vi "WPI_CANTalonSRX_Global.vi"(6 "Set Boolean":bool, 7 "Write After Receive":T2, 8 "Set Number":dbl, 9 "Control Mode":T1, 10 "Operation":T7, 11 "Device ID (0)":u8) -> (1 "Get All":T2, 3 "Device ID Out":u8, 5 "Read For Send":T3={"Output"=0.0, "Control Mode"=enum."Percent VBus", "Brake-Mode Override"=enum."No Override", "Reverse Feedback Sensor"=FALSE, "Reverse Closed-Loop Output"=FALSE, "Override Limits"=FALSE, "Forward Limit Enabled"=FALSE, "Reverse Limit Enabled"=FALSE, "Feedback Select"=0, "Profile Select"=0, "Master To Follow"=0, "Throttle Ramp Rate"=0, "Disabled"=FALSE, "Encoder Codes Per Rev"=0, "Num Pot Turns"=0, "Control Frame Rate Ms"=0, "Use Control5 If Supported"=FALSE, "Enable Frame Rate Ms"=10, "Motion Profile Flow Control"=0, "Motion Profile Control Frame Rate"=10, "Talon SRX Motion Profile Trajectory Point"={"Duration Ms"=0, "Velocity"=0.0, "Position"=0.0, "Profile Slot Select"=0, "Is Last"=FALSE, "Velocity Only"=FALSE, "Zero Position"=FALSE, "Compress Code"=0, "Same Velocity"=0, "Delta Position"=0, "Count"=0}, "Current Limit Enabled"=FALSE} {"Feedback Select" items=["Digital Quadrature Encoder"=0, "Analog Pot"=2, "Analog Encoder"=3, "Count on Quad-A (Rising-Edge)"=4, "Count on Quad-A (Falling-Edge)"=5, "Position is Pulse-Width"=8, "CTR Magnetic Enc (Relative)"=6, "CTR Magnetic Enc (Absolute)"=7]})   [LabVIEW 2016]
uses:
  WPI_CANTalonSRX_GlobalOps.ctl
  WPI_CANTalonSRX_GlobalControl.ctl
  WPI_CANTalonSRX_APIControlMode.ctl
  WPI_CANTalonSRX_BrakeOverride.ctl
  WPI_CANTalonSRX_FeedbackSelect.ctl
  WPI_CANTalonSRX_MotionProfileTrajectoryPt.ctl
  WPI_CANTalonSRX_GlobalStatus.ctl
  WPI_CANTalonSRX_MessageIDs.ctl
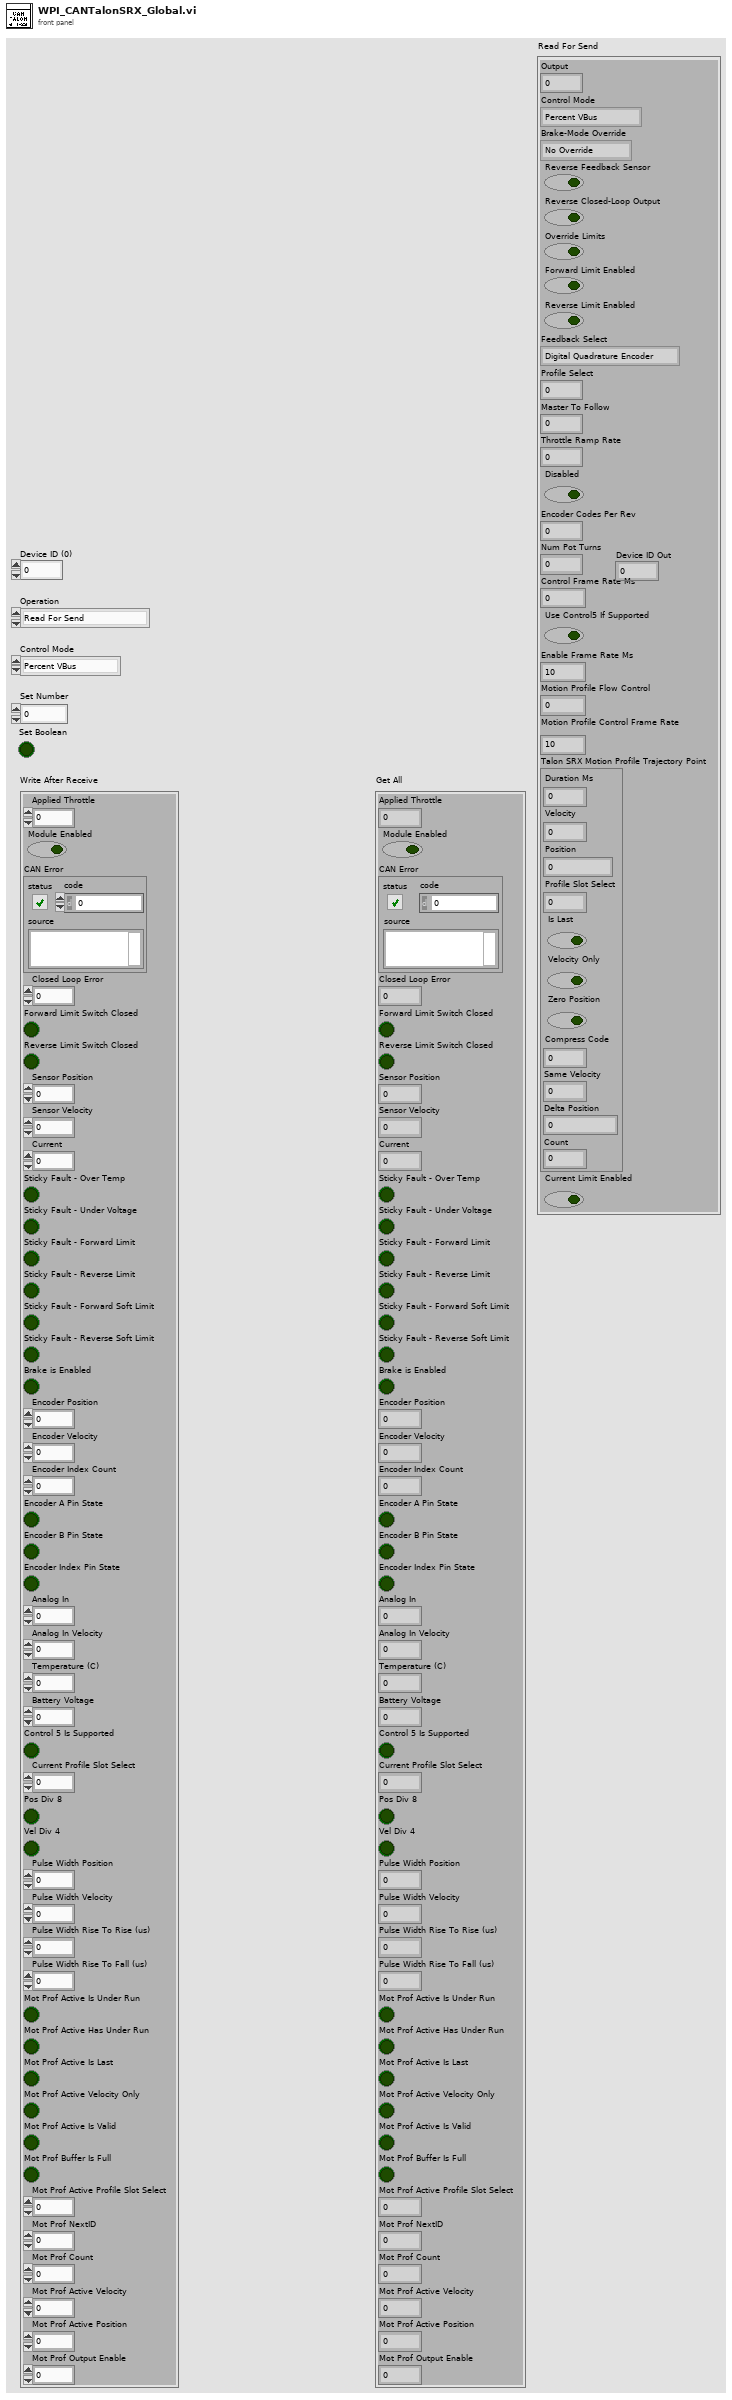
[diagram p1: front panel]
types:
  T1 = typedef "WPI_CANTalonSRX_APIControlMode.ctl" = enum8{"Percent VBus", "Speed", "Position", "Slave", "Unchanged / Invalid", "Voltage Compensation", "Current", "Motion Profile", "Motion Magic"}
  T2 = typedef "WPI_CANTalonSRX_GlobalStatus.ctl" = cluster{"Applied Throttle":dbl, "Module Enabled":bool, "CAN Error":errorcluster, "Closed Loop Error":dbl, "Forward Limit Switch Closed":bool, "Reverse Limit Switch Closed":bool, "Sensor Position":dbl, "Sensor Velocity":dbl, "Current":dbl, "Sticky Fault - Over Temp":bool, "Sticky Fault - Under Voltage":bool, "Sticky Fault - Forward Limit":bool, "Sticky Fault - Reverse Limit":bool, "Sticky Fault - Forward Soft Limit":bool, "Sticky Fault - Reverse Soft Limit":bool, "Brake is Enabled":bool, "Encoder Position":dbl, "Encoder Velocity":dbl, "Encoder Index Count":dbl, "Encoder A Pin State":bool, "Encoder B Pin State":bool, "Encoder Index Pin State":bool, "Analog In":dbl, "Analog In Velocity":dbl, "Temperature (C)":dbl, "Battery Voltage":dbl, "Control 5 Is Supported":bool, "Current Profile Slot Select":dbl, "Pos Div 8":bool, "Vel Div 4":bool, "Pulse Width Position":i32, "Pulse Width Velocity":i32, "Pulse Width Rise To Rise (us)":i32, "Pulse Width Rise To Fall (us)":i32, "Mot Prof Active Is Under Run":bool, "Mot Prof Active Has Under Run":bool, "Mot Prof Active Is Last":bool, "Mot Prof Active Velocity Only":bool, "Mot Prof Active Is Valid":bool, "Mot Prof Buffer Is Full":bool, "Mot Prof Active Profile Slot Select":i32, "Mot Prof NextID":i32, "Mot Prof Count":i32, "Mot Prof Active Velocity":dbl, "Mot Prof Active Position":dbl, "Mot Prof Output Enable":i32}
  T3 = typedef "WPI_CANTalonSRX_GlobalControl.ctl" = cluster{"Output":dbl, "Control Mode":T1, "Brake-Mode Override":T4, "Reverse Feedback Sensor":bool, "Reverse Closed-Loop Output":bool, "Override Limits":bool, "Forward Limit Enabled":bool, "Reverse Limit Enabled":bool, "Feedback Select":T5, "Profile Select":u8, "Master To Follow":u8, "Throttle Ramp Rate":u8, "Disabled":bool, "Encoder Codes Per Rev":u32, "Num Pot Turns":u32, "Control Frame Rate Ms":u8, "Use Control5 If Supported":bool, "Enable Frame Rate Ms":u8, "Motion Profile Flow Control":u8, "Motion Profile Control Frame Rate":u8, "Talon SRX Motion Profile Trajectory Point":T6, "Current Limit Enabled":bool}
  T4 = typedef "WPI_CANTalonSRX_BrakeOverride.ctl" = enum8{"No Override", "Override to Coast", "Override to Brake"}
  T5 = typedef "WPI_CANTalonSRX_FeedbackSelect.ctl" = u8
  T6 = typedef "WPI_CANTalonSRX_MotionProfileTrajectoryPt.ctl" = cluster{"Duration Ms":u8, "Velocity":dbl, "Position":dbl, "Profile Slot Select":u8, "Is Last":bool, "Velocity Only":bool, "Zero Position":bool, "Compress Code":u8, "Same Velocity":i32, "Delta Position":i32, "Count":u8}
  T7 = typedef "WPI_CANTalonSRX_GlobalOps.ctl" = enum16{"Read For Send", "Write After Receive General", "Write After Receive Feedback", "Write After Receive Encoder", "Write After Receive Ain", "Write Error", "Get All", "Set Output", "Set Mode", "Set Master ID", "Set Brake Mode", "Set Reverse Feedback Sensor", "Set Reverse Closed Loop Output", "Set Override Limits", "Set Forward Limit Enabled", "Set Reverse Limit Enabled", "Set Feedback Select", "Set Profile Select", "Set Throttle Ramp Rate", "Disable", "Set Enc Codes Per Rev", "Set Num Pot Turns", "Set Control Frame Rate", "Enable Legacy Control", "Write After Receive Pulse Width", "Set Enable Frame Rate", "Write After Receive Motion Profile", "Set Motion Profile Flow Control", "Set Motion Profile Control Frame Rate", "Set Current Limit Enable"}
  T8 = typedef "WPI_CANTalonSRX_MessageIDs.ctl" = u32
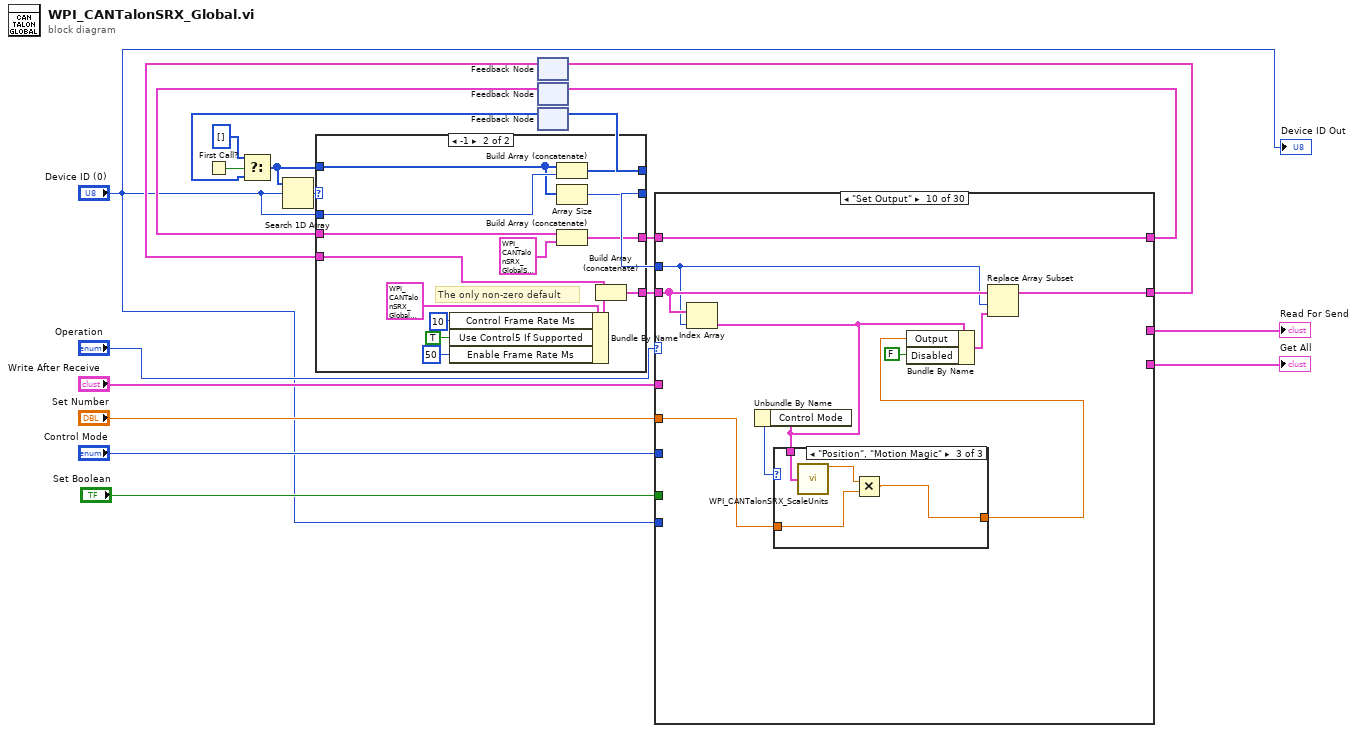
[diagram p0: block diagram]
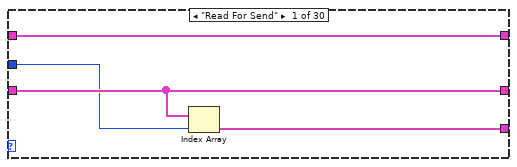
[diagram p2: hidden frame]
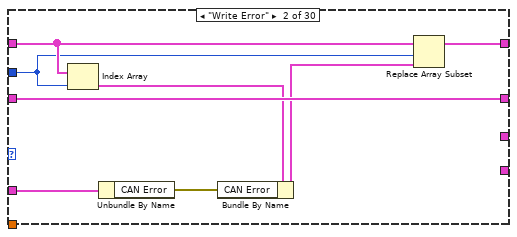
[diagram p3: hidden frame]
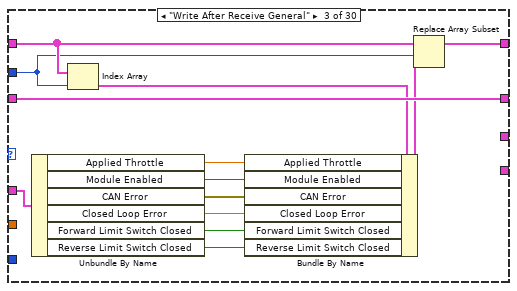
[diagram p4: hidden frame]
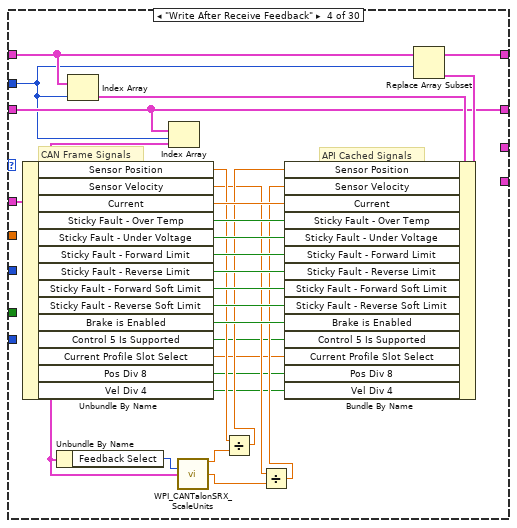
[diagram p5: hidden frame]
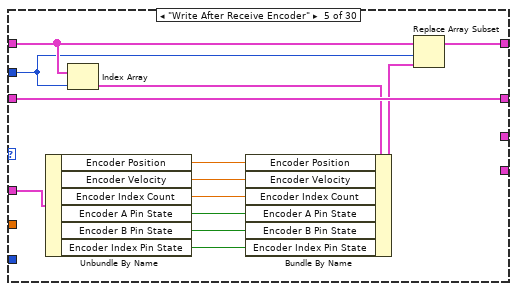
[diagram p6: hidden frame]
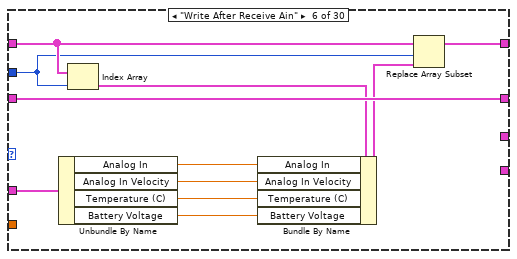
[diagram p7: hidden frame]
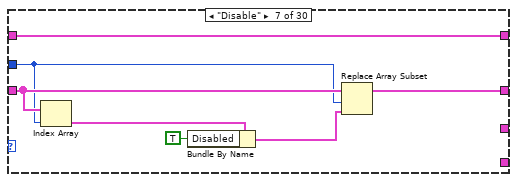
[diagram p8: hidden frame]
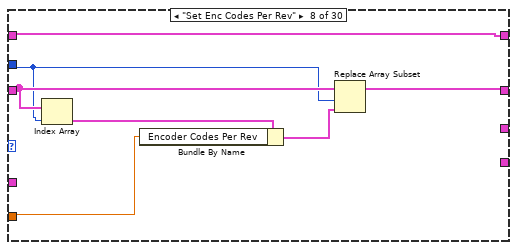
[diagram p9: hidden frame]
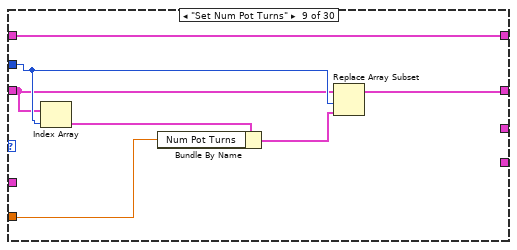
[diagram p10: hidden frame]
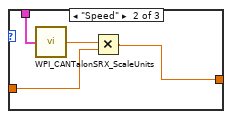
[diagram p12: hidden frame]
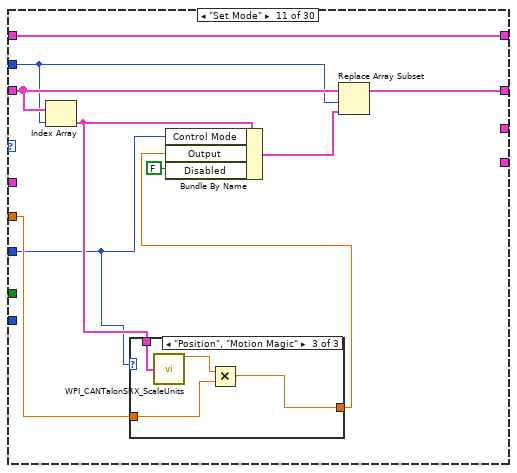
[diagram p13: hidden frame]
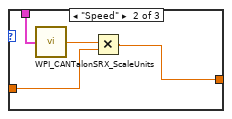
[diagram p15: hidden frame]
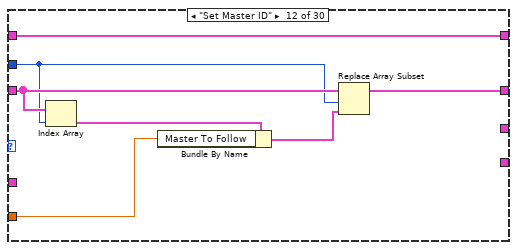
[diagram p16: hidden frame]
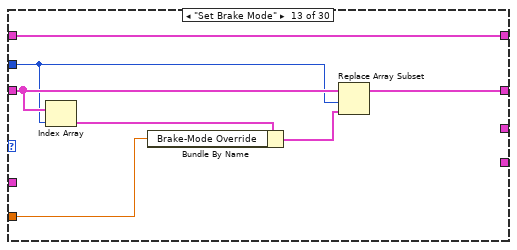
[diagram p17: hidden frame]
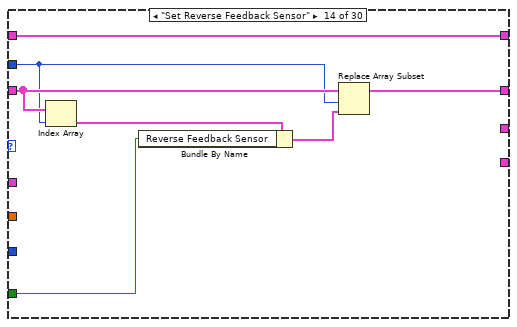
[diagram p18: hidden frame]
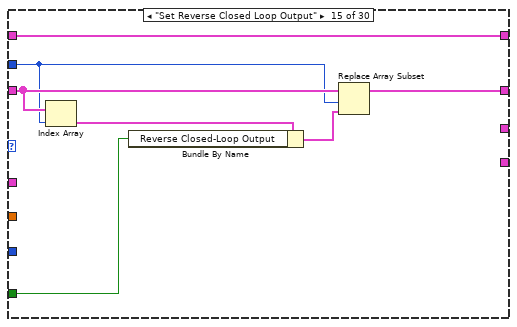
[diagram p19: hidden frame]
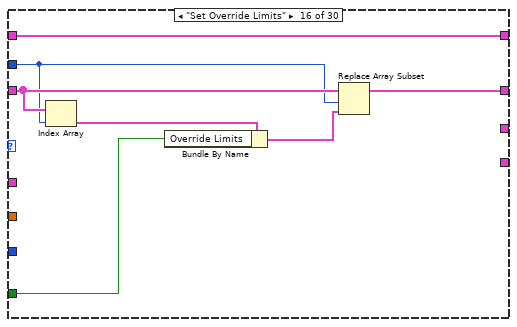
[diagram p20: hidden frame]
diagram:
  n1 = First Call?() -> (First Call?: T/F=w21:bool)
  n2 = feedback #1() -> (w14:T3[])  [unwired: 1 in]
  n3 = feedback #2() -> (w15:T2[])  [unwired: 1 in]
  n4 = feedback #3() -> (w19:u8[])  [unwired: 1 in]
  n5 = Select(t=u8[] [], s=w21, f=w19) -> (s? t:f=w17:u8[])
  n6 = Search 1D Array(1D array=w17, element="Device ID (0)") -> (index of element=w16:i32)  [unwired: 1 in]
  n7 = case shown="-1" w16 {
    selector: w16 -> [w22 _]
    tunnel: [w25 w39] -> w18
    tunnel: "Device ID (0)" -> [_ w38]
    tunnel: w17 -> [w25 w33]
    tunnel: w15 -> [w24 w37]
    tunnel: w14 -> [w23 w36]
    tunnel: [w24 w35] -> w12
    tunnel: [w23 w34] -> w10
    tunnel: [w22 w32] -> w9
    frame Default {
    }
    frame -1 {
      # "The only non-zero default"
      n8 = Bundle By Name(cluster=T3 {"Output"=0.0, "Control Mode"=enum."Percent VBus", "Brake-Mode Override"=enum."No Override", "Reverse Feedback Sensor"=FALSE, "Reverse Closed-Loop Output"=FALSE, "Override Limits"=FALSE, "Forward Limit Enabled"=FALSE, "Reverse Limit Enabled"=FALSE, "Feedback Select"=0, "Profile Select"=0, "Master To Follow"=0, "Throttle Ramp Rate"=0, "Disabled"=FALSE, "Encoder Codes Per Rev"=0, "Num Pot Turns"=0, "Control Frame Rate Ms"=0, "Use Control5 If Supported"=FALSE, "Enable Frame Rate Ms"=10, "Motion Profile Flow Control"=0, "Motion Profile Control Frame Rate"=10, "Talon SRX Motion Profile Trajectory Point"={"Duration Ms"=0, "Velocity"=0.0, "Position"=0.0, "Profile Slot Select"=0, "Is Last"=FALSE, "Velocity Only"=FALSE, "Zero Position"=FALSE, "Compress Code"=0, "Same Velocity"=0, "Delta Position"=0, "Count"=0}, "Current Limit Enabled"=FALSE} ("Read For Send"), "Control Frame Rate Ms"=u8 10, "Use Control5 If Supported"=TRUE, "Enable Frame Rate Ms"=u8 50) -> (w30:T3)
      n9 = Build Array (concatenate)(w33, w38) -> (w39:u8[])
      n10 = Array Size(array=w33) -> (size(s)=w32:i32)
      n11 = Build Array (concatenate)(w37, T2 {"Applied Throttle"=0.0, "Module Enabled"=FALSE, "CAN Error"={"status"=FALSE, "code"=0, "source"=""}, "Closed Loop Error"=0.0, "Forward Limit Switch Closed"=FALSE, "Reverse Limit Switch Closed"=FALSE, "Sensor Position"=0.0, "Sensor Velocity"=0.0, "Current"=0.0, "Sticky Fault - Over Temp"=FALSE, "Sticky Fault - Under Voltage"=FALSE, "Sticky Fault - Forward Limit"=FALSE, "Sticky Fault - Reverse Limit"=FALSE, "Sticky Fault - Forward Soft Limit"=FALSE, "Sticky Fault - Reverse Soft Limit"=FALSE, "Brake is Enabled"=FALSE, "Encoder Position"=0.0, "Encoder Velocity"=0.0, "Encoder Index Count"=0.0, "Encoder A Pin State"=FALSE, "Encoder B Pin State"=FALSE, "Encoder Index Pin State"=FALSE, "Analog In"=0.0, "Analog In Velocity"=0.0, "Temperature (C)"=0.0, "Battery Voltage"=0.0, "Control 5 Is Supported"=FALSE, "Current Profile Slot Select"=0.0, "Pos Div 8"=FALSE, "Vel Div 4"=FALSE, "Pulse Width Position"=0, "Pulse Width Velocity"=0, "Pulse Width Rise To Rise (us)"=0, "Pulse Width Rise To Fall (us)"=0, "Mot Prof Active Is Under Run"=FALSE, "Mot Prof Active Has Under Run"=FALSE, "Mot Prof Active Is Last"=FALSE, "Mot Prof Active Velocity Only"=FALSE, "Mot Prof Active Is Valid"=FALSE, "Mot Prof Buffer Is Full"=FALSE, "Mot Prof Active Profile Slot Select"=0, "Mot Prof NextID"=0, "Mot Prof Count"=0, "Mot Prof Active Velocity"=0.0, "Mot Prof Active Position"=0.0, "Mot Prof Output Enable"=0} ("Write After Receive")) -> (w35:T2[])
      n12 = Build Array (concatenate)(w36, w30) -> (w34:T3[])
    }
  }
  n13 = feedback-in #3(w18) -> ()
  n14 = case shown="\"Set Output\"" "Operation" {
    tunnel: [w43 w50 w63 w91 w103 w114 w122 w128 w130 w146 w161 w176 w183 w190 w197 w204 w211 w218 w225 w232 w239 w246 w252 w264 w273 w283 w306 w320 w324 w335] -> w13
    tunnel: w12 -> [w43 w49 w62 w90 w102 w113 w122 w128 w130 w146 w161 w176 w183 w190 w197 w204 w211 w218 w225 w232 w239 w246 w252 w264 w274 w283 w307 w320 w324 w335]
    tunnel: [w42 w51 w64 w78 w104 w115 w120 w125 w133 w144 w165 w181 w188 w195 w202 w209 w216 w223 w230 w237 w244 w248 w254 w261 w272 w282 w296 w319 w323 w332] -> w11
    tunnel: w10 -> [w42 w51 w64 w78 w104 w115 w121 w127 w131 w145 w164 w180 w187 w194 w201 w208 w215 w222 w229 w236 w243 w248 w255 w262 w272 w284 w296 w317 w326 w333]
    tunnel: w9 -> [w41 w48 w61 w77 w101 w112 w119 w124 w132 w143 w163 w179 w186 w193 w200 w207 w214 w221 w228 w235 w242 w247 w253 w263 w275 w285 w295 w321 w325 w334]
    tunnel: [w40 _ _ _ _ _ _ _ _ _ _ _ _ _ _ _ _ _ _ _ _ _ _ _ _ _ _ _ _ _] -> w8
    tunnel: "Write After Receive" -> [_ w45 w60 w89 w100 w111 _ _ _ _ _ _ _ _ _ _ _ _ _ _ _ _ _ _ w271 _ w308 _ _ _]
    tunnel: "Set Number" -> [_ _ _ _ _ _ _ w126 w134 w139 w159 w175 w182 _ _ _ _ _ w224 w231 w238 _ w250 _ _ w286 _ w316 w327 _]
    tunnel: [_ _ _ _ _ _ _ _ _ _ _ _ _ _ _ _ _ _ _ _ _ w245 _ _ _ _ _ _ _ _] -> w5
    tunnel: "Control Mode" -> [_ _ _ _ _ _ _ _ _ _ w156 _ _ _ _ _ _ _ _ _ _ _ _ _ _ _ _ _ _ _]
    tunnel: "Set Boolean" -> [_ _ _ _ _ _ _ _ _ _ _ _ _ w189 w196 w203 w210 w217 _ _ _ _ _ w258 _ _ _ _ _ w331]
    tunnel: "Device ID (0)" -> [_ _ _ _ _ _ _ _ _ _ _ _ _ _ _ _ _ _ _ _ _ _ _ w259 _ _ _ _ _ _]
    frame "Read For Send" {
      n15 = Index Array(array=w42, index=w41) -> (element=w40:T3)
    }
    frame "Write Error" {
      n16 = Index Array(array=w49, index=w48) -> (element=w47:T2)
      n17 = Unbundle By Name(w45) -> ("CAN Error"=w44:errorcluster)
      n18 = Bundle By Name(cluster=w47, "CAN Error"=w44) -> (w46:T2)
      n19 = Replace Array Subset(array=w49, new element=w46, index=w48) -> (w50:T2[])
    }
    frame "Write After Receive General" {
      n20 = Unbundle By Name(w60) -> ("Applied Throttle"=w57:dbl, "Module Enabled"=w56:bool, "CAN Error"=w55:errorcluster, "Closed Loop Error"=w54:dbl, "Forward Limit Switch Closed"=w53:bool, "Reverse Limit Switch Closed"=w52:bool)
      n21 = Index Array(array=w62, index=w61) -> (element=w59:T2)
      n22 = Bundle By Name(cluster=w59, "Applied Throttle"=w57, "Module Enabled"=w56, "CAN Error"=w55, "Closed Loop Error"=w54, "Forward Limit Switch Closed"=w53, "Reverse Limit Switch Closed"=w52) -> (w58:T2)
      n23 = Replace Array Subset(array=w62, new element=w58, index=w61) -> (w63:T2[])
    }
    frame "Write After Receive Feedback" {
      # "API Cached Signals"
      # "CAN Frame Signals"
      n24 = Unbundle By Name(w89) -> ("Sensor Position"=w75:dbl, "Sensor Velocity"=w73:dbl, "Current"=w86:dbl, "Sticky Fault - Over Temp"=w85:bool, "Sticky Fault - Under Voltage"=w84:bool, "Sticky Fault - Forward Limit"=w83:bool, "Sticky Fault - Reverse Limit"=w79:bool, "Sticky Fault - Forward Soft Limit"=w80:bool, "Sticky Fault - Reverse Soft Limit"=w81:bool, "Brake is Enabled"=w82:bool, "Control 5 Is Supported"=w65:bool, "Current Profile Slot Select"=w66:dbl, "Pos Div 8"=w67:bool, "Vel Div 4"=w68:bool)
      n25 = Index Array(array=w90, index=w77) -> (element=w88:T2)
      n26 = Index Array(array=w78, index=w77) -> (element=w70:T3)
      n27 = Unbundle By Name(w70) -> ("Feedback Select"=w69:T5)
      n28 = call "WPI_CANTalonSRX_ScaleUnits.vi"("Feedback Scalar Select"=w69, "Read For Send"=w70) -> ("Position Scalar"=w74:dbl, "Velocity Scalar"=w72:dbl)  [unwired: 11 in, 1 out]
      n29 = Divide(x=w75, y=w74) -> (x/y=w76:dbl)
      n30 = Divide(x=w73, y=w72) -> (x/y=w71:dbl)
      n31 = Bundle By Name(cluster=w88, "Sensor Position"=w76, "Sensor Velocity"=w71, "Current"=w86, "Sticky Fault - Over Temp"=w85, "Sticky Fault - Under Voltage"=w84, "Sticky Fault - Forward Limit"=w83, "Sticky Fault - Reverse Limit"=w79, "Sticky Fault - Forward Soft Limit"=w80, "Sticky Fault - Reverse Soft Limit"=w81, "Brake is Enabled"=w82, "Control 5 Is Supported"=w65, "Current Profile Slot Select"=w66, "Pos Div 8"=w67, "Vel Div 4"=w68) -> (w87:T2)
      n32 = Replace Array Subset(array=w90, new element=w87, index=w77) -> (w91:T2[])
    }
    frame "Write After Receive Encoder" {
      n33 = Unbundle By Name(w100) -> ("Encoder Position"=w97:dbl, "Encoder Velocity"=w96:dbl, "Encoder Index Count"=w95:dbl, "Encoder A Pin State"=w94:bool, "Encoder B Pin State"=w93:bool, "Encoder Index Pin State"=w92:bool)
      n34 = Index Array(array=w102, index=w101) -> (element=w99:T2)
      n35 = Bundle By Name(cluster=w99, "Encoder Position"=w97, "Encoder Velocity"=w96, "Encoder Index Count"=w95, "Encoder A Pin State"=w94, "Encoder B Pin State"=w93, "Encoder Index Pin State"=w92) -> (w98:T2)
      n36 = Replace Array Subset(array=w102, new element=w98, index=w101) -> (w103:T2[])
    }
    frame "Write After Receive Ain" {
      n37 = Unbundle By Name(w111) -> ("Analog In"=w108:dbl, "Analog In Velocity"=w107:dbl, "Temperature (C)"=w106:dbl, "Battery Voltage"=w105:dbl)
      n38 = Index Array(array=w113, index=w112) -> (element=w110:T2)
      n39 = Bundle By Name(cluster=w110, "Analog In"=w108, "Analog In Velocity"=w107, "Temperature (C)"=w106, "Battery Voltage"=w105) -> (w109:T2)
      n40 = Replace Array Subset(array=w113, new element=w109, index=w112) -> (w114:T2[])
    }
    frame "Disable" {
      n41 = Index Array(array=w121, index=w119) -> (element=w118:T3)
      n42 = Bundle By Name(cluster=w118, "Disabled"=TRUE) -> (w117:T3)
      n43 = Replace Array Subset(array=w121, new element=w117, index=w119) -> (w120:T3[])
    }
    frame "Set Enc Codes Per Rev" {
      n44 = Index Array(array=w127, index=w124) -> (element=w123:T3)
      n45 = Bundle By Name(cluster=w123, "Encoder Codes Per Rev"=w126) -> (w129:T3)
      n46 = Replace Array Subset(array=w127, new element=w129, index=w124) -> (w125:T3[])
    }
    frame "Set Num Pot Turns" {
      n47 = Index Array(array=w131, index=w132) -> (element=w135:T3)
      n48 = Bundle By Name(cluster=w135, "Num Pot Turns"=w134) -> (w136:T3)
      n49 = Replace Array Subset(array=w131, new element=w136, index=w132) -> (w133:T3[])
    }
    frame "Set Output" {
      n50 = Index Array(array=w145, index=w143) -> (element=w137:T3)
      n51 = Unbundle By Name(w137) -> ("Control Mode"=w140:T1)
      n52 = case shown="\"Position\", \"Motion Magic\"" w140 {
        tunnel: [w147 w148 w154] -> w138
        tunnel: w139 -> [w147 w150 w152]
        tunnel: w137 -> [_ w151 w155]
        frame Default {
        }
        frame "Speed" {
          n53 = call "WPI_CANTalonSRX_ScaleUnits.vi"("Read For Send"=w151) -> ("Velocity Scalar"=w149:dbl)  [unwired: 12 in, 2 out]
          n54 = Multiply(x=w149, y=w150) -> (x*y=w148:dbl)
        }
        frame "Position", "Motion Magic" {
          n55 = call "WPI_CANTalonSRX_ScaleUnits.vi"("Read For Send"=w155) -> ("Position Scalar"=w153:dbl)  [unwired: 12 in, 2 out]
          n56 = Multiply(x=w153, y=w152) -> (x*y=w154:dbl)
        }
      }
      n57 = Bundle By Name(cluster=w137, "Output"=w138, "Disabled"=FALSE) -> (w142:T3)
      n58 = Replace Array Subset(array=w145, new element=w142, index=w143) -> (w144:T3[])
    }
    frame "Set Mode" {
      n59 = Index Array(array=w164, index=w163) -> (element=w157:T3)
      n60 = case shown="\"Position\", \"Motion Magic\"" w156 {
        tunnel: [w166 w167 w173] -> w158
        tunnel: w159 -> [w166 w169 w171]
        tunnel: w157 -> [_ w170 w174]
        frame Default {
        }
        frame "Speed" {
          n61 = call "WPI_CANTalonSRX_ScaleUnits.vi"("Read For Send"=w170) -> ("Velocity Scalar"=w168:dbl)  [unwired: 12 in, 2 out]
          n62 = Multiply(x=w168, y=w169) -> (x*y=w167:dbl)
        }
        frame "Position", "Motion Magic" {
          n63 = call "WPI_CANTalonSRX_ScaleUnits.vi"("Read For Send"=w174) -> ("Position Scalar"=w172:dbl)  [unwired: 12 in, 2 out]
          n64 = Multiply(x=w172, y=w171) -> (x*y=w173:dbl)
        }
      }
      n65 = Bundle By Name(cluster=w157, "Control Mode"=w156, "Output"=w158, "Disabled"=FALSE) -> (w162:T3)
      n66 = Replace Array Subset(array=w164, new element=w162, index=w163) -> (w165:T3[])
    }
    frame "Set Master ID" {
      n67 = Index Array(array=w180, index=w179) -> (element=w178:T3)
      n68 = Bundle By Name(cluster=w178, "Master To Follow"=w175) -> (w177:T3)
      n69 = Replace Array Subset(array=w180, new element=w177, index=w179) -> (w181:T3[])
    }
    frame "Set Brake Mode" {
      n70 = Index Array(array=w187, index=w186) -> (element=w185:T3)
      n71 = Bundle By Name(cluster=w185, "Brake-Mode Override"=w182) -> (w184:T3)
      n72 = Replace Array Subset(array=w187, new element=w184, index=w186) -> (w188:T3[])
    }
    frame "Set Reverse Feedback Sensor" {
      n73 = Index Array(array=w194, index=w193) -> (element=w192:T3)
      n74 = Bundle By Name(cluster=w192, "Reverse Feedback Sensor"=w189) -> (w191:T3)
      n75 = Replace Array Subset(array=w194, new element=w191, index=w193) -> (w195:T3[])
    }
    frame "Set Reverse Closed Loop Output" {
      n76 = Index Array(array=w201, index=w200) -> (element=w199:T3)
      n77 = Bundle By Name(cluster=w199, "Reverse Closed-Loop Output"=w196) -> (w198:T3)
      n78 = Replace Array Subset(array=w201, new element=w198, index=w200) -> (w202:T3[])
    }
    frame "Set Override Limits" {
      n79 = Index Array(array=w208, index=w207) -> (element=w206:T3)
      n80 = Bundle By Name(cluster=w206, "Override Limits"=w203) -> (w205:T3)
      n81 = Replace Array Subset(array=w208, new element=w205, index=w207) -> (w209:T3[])
    }
    frame "Set Forward Limit Enabled" {
      n82 = Index Array(array=w215, index=w214) -> (element=w213:T3)
      n83 = Bundle By Name(cluster=w213, "Forward Limit Enabled"=w210) -> (w212:T3)
      n84 = Replace Array Subset(array=w215, new element=w212, index=w214) -> (w216:T3[])
    }
    frame "Set Reverse Limit Enabled" {
      n85 = Index Array(array=w222, index=w221) -> (element=w220:T3)
      n86 = Bundle By Name(cluster=w220, "Reverse Limit Enabled"=w217) -> (w219:T3)
      n87 = Replace Array Subset(array=w222, new element=w219, index=w221) -> (w223:T3[])
    }
    frame "Set Feedback Select" {
      n88 = Index Array(array=w229, index=w228) -> (element=w227:T3)
      n89 = Bundle By Name(cluster=w227, "Feedback Select"=w224) -> (w226:T3)
      n90 = Replace Array Subset(array=w229, new element=w226, index=w228) -> (w230:T3[])
    }
    frame "Set Profile Select" {
      n91 = Index Array(array=w236, index=w235) -> (element=w234:T3)
      n92 = Bundle By Name(cluster=w234, "Profile Select"=w231) -> (w233:T3)
      n93 = Replace Array Subset(array=w236, new element=w233, index=w235) -> (w237:T3[])
    }
    frame "Set Throttle Ramp Rate" {
      n94 = Index Array(array=w243, index=w242) -> (element=w241:T3)
      n95 = Bundle By Name(cluster=w241, "Throttle Ramp Rate"=w238) -> (w240:T3)
      n96 = Replace Array Subset(array=w243, new element=w240, index=w242) -> (w244:T3[])
    }
    frame "Get All" {
      n97 = Index Array(array=w246, index=w247) -> (element=w245:T2)
    }
    frame "Set Control Frame Rate" {
      n98 = Index Array(array=w255, index=w253) -> (element=w251:T3)
      n99 = To Unsigned Byte Integer(number=w250) -> (unsigned 8bit integer=w249:u8)
      n100 = Bundle By Name(cluster=w251, "Control Frame Rate Ms"=w249) -> (w256:T3)
      n101 = Replace Array Subset(array=w255, new element=w256, index=w253) -> (w254:T3[])
    }
    frame "Enable Legacy Control" {
      n102 = Index Array(array=w262, index=w263) -> (element=w265:T3)
      n103 = case shown="True" w258 {
        tunnel: w259 -> [_ w266]
        frame False {
        }
        frame True {
          w267 = T8 33816832 items=["TalonSRX Control General 10ms"=33816576, "TalonSRX Control Rates Slow"=33816640, "TalonSRX Control ClearFlags Slow"=33816704, "TalonSRX Status General 10ms"=33821696, "TalonSRX Status Feedback 20ms"=33821760, "TalonSRX Status Enc 100ms"=33821824, "TalonSRX Status AinTempVbat 100ms"=33821888, "TalonSRX Status Startup Once"=33821952, "TalonSRX Status Debug"=33822080, "TalonSRX Config SetGainsSlot0 A"=33823808, "TalonSRX Config SetGainsSlot0 B"=33823872, "TalonSRX Config SetGainsSlot1 A"=33823936, "TalonSRX Config SetGainsSlot1 B"=33824000, "TalonSRX Config SetSoftLimits"=33824064, "TalonSRX Config WebControl"=33824128, "TalonSRX Param Request"=33822720, "TalonSRX Param Response"=33822784, "TalonSRX Param Set"=33822848, "TalonSRX Status PulseWidth"=33822144, "TalonSRX Status Motion Profile"=33822208, "TalonSRX Control General 5"=33816832, "TalonSRX Control Motion Profile Add"=33816896] ("Talon SRX Control Frame")
          # "Turn off Control 5, Send VI will use Control 1"
          n104 = Or(x=w266, y=w267) -> (x .or. y?=w268:T8)
          n105 = call <vilib>:"NetComm_CAN_Send.vi"("Period (ms)"=0, "Data"=u8[] [] ("Token Space"), "Message ID"=w268) -> ()  [unwired: 8 in, 1 out]
        }
      }
      n106 = Not(x=w258) -> (.not. x?=w260:bool)
      n107 = Bundle By Name(cluster=w265, "Use Control5 If Supported"=w260) -> (w257:T3)
      n108 = Replace Array Subset(array=w262, new element=w257, index=w263) -> (w261:T3[])
    }
    frame "Write After Receive Pulse Width" {
      n109 = Unbundle By Name(w271) -> ("Pulse Width Position"=w279:i32, "Pulse Width Velocity"=w278:i32, "Pulse Width Rise To Rise (us)"=w277:i32, "Pulse Width Rise To Fall (us)"=w276:i32)
      n110 = Index Array(array=w274, index=w275) -> (element=w281:T2)
      n111 = Bundle By Name(cluster=w281, "Pulse Width Position"=w279, "Pulse Width Velocity"=w278, "Pulse Width Rise To Rise (us)"=w277, "Pulse Width Rise To Fall (us)"=w276) -> (w280:T2)
      n112 = Replace Array Subset(array=w274, new element=w280, index=w275) -> (w273:T2[])
    }
    frame "Set Enable Frame Rate" {
      n113 = Index Array(array=w284, index=w285) -> (element=w288:T3)
      n114 = To Unsigned Byte Integer(number=w286) -> (unsigned 8bit integer=w287:u8)
      n115 = Bundle By Name(cluster=w288, "Enable Frame Rate Ms"=w287) -> (w289:T3)
      n116 = Replace Array Subset(array=w284, new element=w289, index=w285) -> (w282:T3[])
    }
    frame "Write After Receive Motion Profile" {
      # "API Cached Signals"
      # "CAN Frame Signals"
      n117 = Unbundle By Name(w308) -> ("Mot Prof Active Is Under Run"=w312:bool, "Mot Prof Active Has Under Run"=w311:bool, "Mot Prof Active Is Last"=w310:bool, "Mot Prof Active Velocity Only"=w309:bool, "Mot Prof Active Is Valid"=w305:bool, "Mot Prof Buffer Is Full"=w304:bool, "Mot Prof Active Profile Slot Select"=w303:i32, "Mot Prof NextID"=w302:i32, "Mot Prof Count"=w301:i32, "Mot Prof Active Velocity"=w293:dbl, "Mot Prof Active Position"=w291:dbl, "Mot Prof Output Enable"=w300:i32)
      n118 = Index Array(array=w296, index=w295) -> (element=w294:T3)
      n119 = Unbundle By Name(w294) -> ("Feedback Select"=w297:T5)
      n120 = Index Array(array=w307, index=w295) -> (element=w314:T2)
      n121 = call "WPI_CANTalonSRX_ScaleUnits.vi"("Feedback Scalar Select"=w297, "Read For Send"=w294) -> ("Position Scalar"=w299:dbl, "Velocity Scalar"=w298:dbl)  [unwired: 11 in, 1 out]
      n122 = Divide(x=w291, y=w299) -> (x/y=w290:dbl)
      n123 = Divide(x=w293, y=w298) -> (x/y=w292:dbl)
      n124 = Bundle By Name(cluster=w314, "Mot Prof Active Is Under Run"=w312, "Mot Prof Active Has Under Run"=w311, "Mot Prof Active Is Last"=w310, "Mot Prof Active Velocity Only"=w309, "Mot Prof Active Is Valid"=w305, "Mot Prof Buffer Is Full"=w304, "Mot Prof Active Profile Slot Select"=w303, "Mot Prof NextID"=w302, "Mot Prof Count"=w301, "Mot Prof Active Velocity"=w292, "Mot Prof Active Position"=w290, "Mot Prof Output Enable"=w300) -> (w313:T2)
      n125 = Replace Array Subset(array=w307, new element=w313, index=w295) -> (w306:T2[])
    }
    frame "Set Motion Profile Flow Control" {
      n126 = Index Array(array=w317, index=w321) -> (element=w318:T3)
      n127 = To Unsigned Byte Integer(number=w316) -> (unsigned 8bit integer=w315:u8)
      n128 = Bundle By Name(cluster=w318, "Motion Profile Flow Control"=w315) -> (w322:T3)
      n129 = Replace Array Subset(array=w317, new element=w322, index=w321) -> (w319:T3[])
    }
    frame "Set Motion Profile Control Frame Rate" {
      n130 = Index Array(array=w326, index=w325) -> (element=w329:T3)
      n131 = To Unsigned Byte Integer(number=w327) -> (unsigned 8bit integer=w328:u8)
      n132 = Bundle By Name(cluster=w329, "Motion Profile Control Frame Rate"=w328) -> (w330:T3)
      n133 = Replace Array Subset(array=w326, new element=w330, index=w325) -> (w323:T3[])
    }
    frame "Set Current Limit Enable" {
      n134 = Index Array(array=w333, index=w334) -> (element=w337:T3)
      n135 = Bundle By Name(cluster=w337, "Current Limit Enabled"=w331) -> (w336:T3)
      n136 = Replace Array Subset(array=w333, new element=w336, index=w334) -> (w332:T3[])
    }
  }
  "Read For Send" <- w8
  "Get All" <- w5
  n137 = feedback-in #1(w11) -> ()
  n138 = feedback-in #2(w13) -> ()
  "Device ID Out" <- "Device ID (0)"
